vi "Day 7 - No Space Left On Device.vi"() -> ()   [LabVIEW 2020, in "AoC 2022.lvlib"]
uses:
  AoC 2022.lvlib
panel:
  in  "Directory Tree":string(tree)
  out "Puzzle Part-2 Answer":string
  out "Puzzle Answer":string
  in  "Puzzle Input":string="$ cd /\n$ ls\ndir a\n14848514 b.txt\n8504156 c.dat\ndir d\n$ cd a\n$ ls\ndir e\n29116 f\n2557 g\n62596 h.lst\n$ cd e\n$ ls\n584 i\n$ cd ..\n$ cd ..\n$ cd d\n$ ls\n4060174 j\n8033020 d.log\n5626152 d.ext\n7214296 k"
  # "Press Ctrl+M & Enter the Puzzle Input and run the VI"
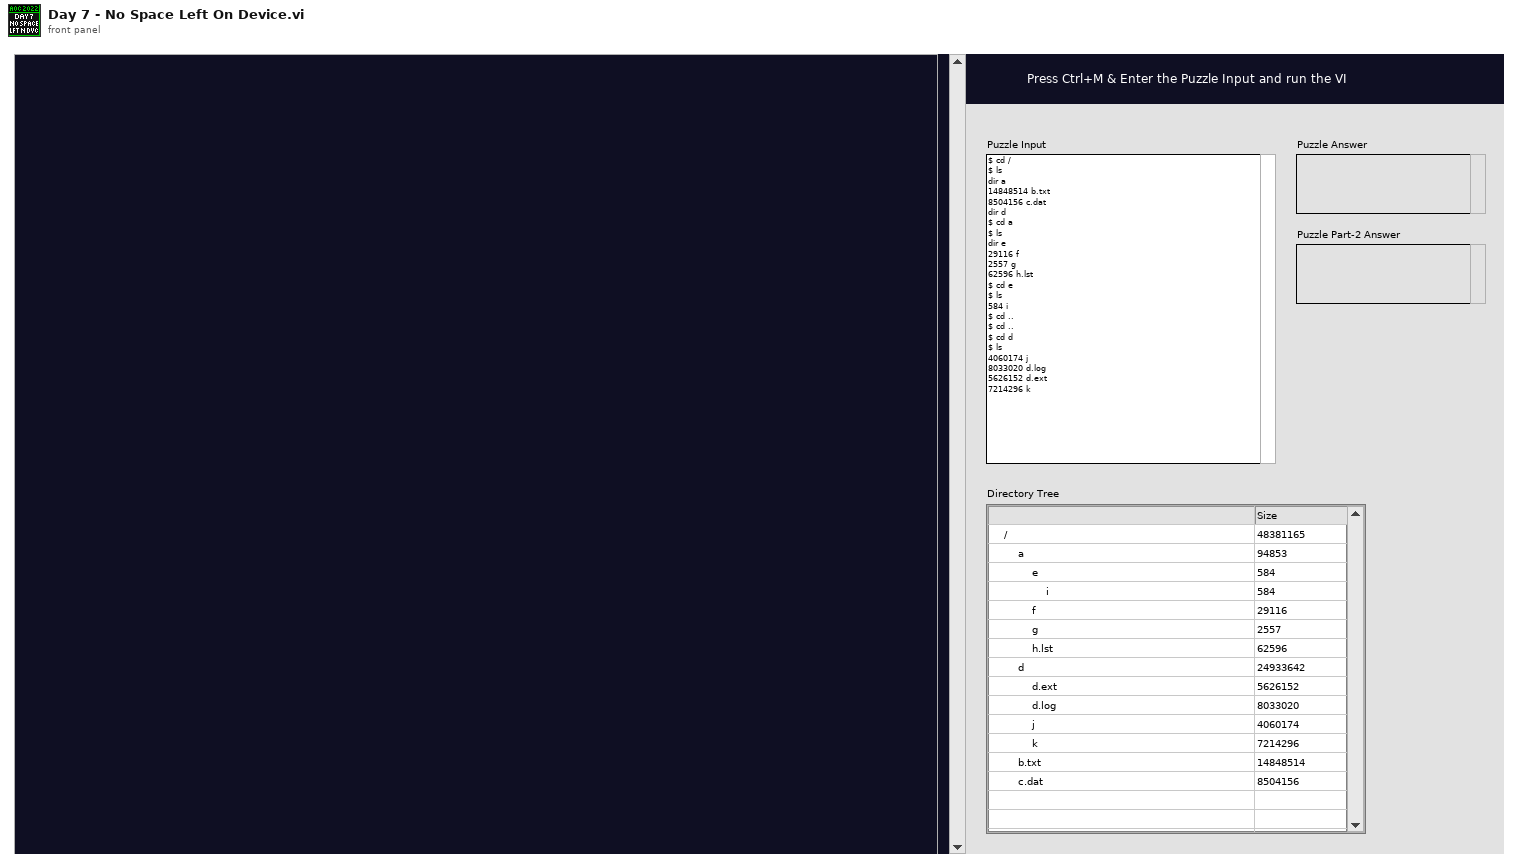
[diagram p1: front panel]
types:
  T1 = typedef "AoC 2022.lvlib/Directory Tree.ctl" = map{string, T2}
  T2 = typedef "AoC 2022.lvlib/Directory Content.ctl" = cluster{"Directories":set{string}, "Files":T3}
  T3 = typedef "AoC 2022.lvlib/File.ctl" = map{string, u64}
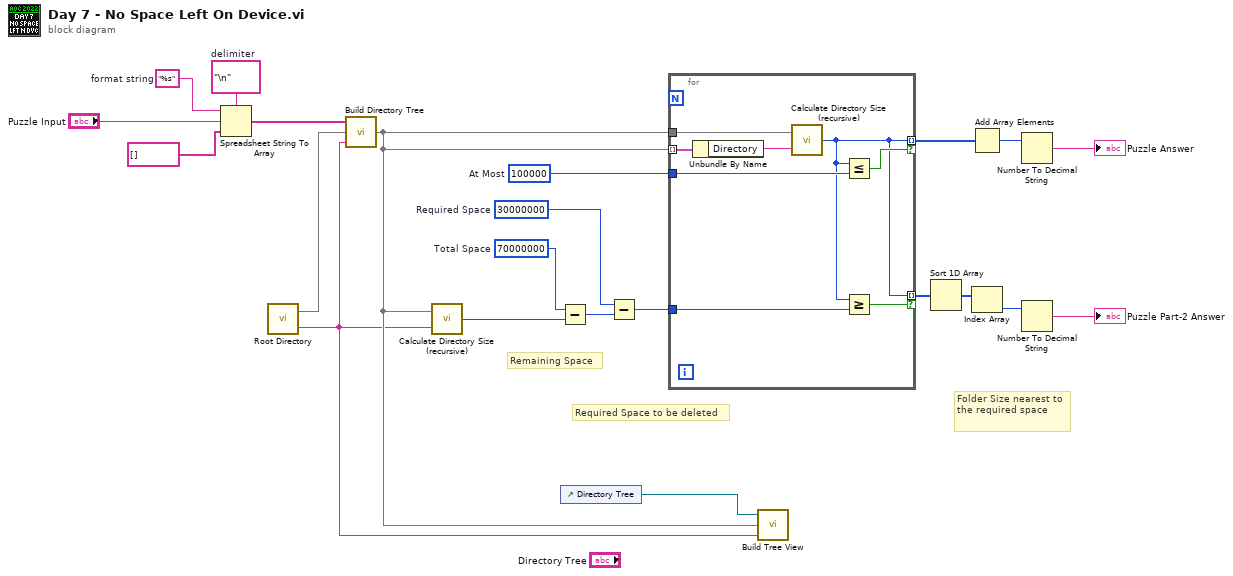
[diagram p0: block diagram]
diagram:
  w8 = u64 30000000  # Required Space
  w10 = u64 70000000  # Total Space
  w14 = u64 100000  # At Most
  w20 = "%s"  # format string
  w22 = "\n"  # delimiter
  # "Folder Size nearest to the required space"
  # "Required Space to be deleted"
  # "Remaining Space"
  n1 = Spreadsheet String To Array(delimiter (Tab)=w22, format string=w20, spreadsheet string="Puzzle Input", array type (2D Dbl)=string[] []) -> (array=w15:string[])
  n2 = call "Root Directory.vi"() -> ("Root Directory"=w1:string, "Directory Tree"=w16:T1)
  n3 = call "Build Directory Tree.vi"("Root Directory"=w1, "Directory Tree in"=w16, "Printed Data on Terminal"=w15) -> ("Directory Tree out"=w2:T1)  [unwired: 2 in]
  n4 = call "Calculate Directory Size (recursive).vi"("Directory"=w1, "Directory Tree"=w2) -> ("Directory Size"=w9:u64)
  n5 = Subtract(x=w10, y=w9) -> (x-y=w7:u64)
  n6 = control-ref of="Directory Tree"() -> (w3:refnum<vi>)
  n7 = Subtract(x=w8, y=w7) -> (x-y=w6:u64)
  n8 = for {
    tunnel: w2 -> [w30] mode=indexing
    tunnel: w2 -> [w28]
    tunnel: [w24] -> w11 mode=indexing if=w27
    tunnel: w14 -> [w26]
    tunnel: w6 -> [w25]
    tunnel: [w24] -> w5 mode=indexing if=w23
    n9 = Unbundle By Name(w30) -> ("Directory"=w29:string)
    n10 = call "Calculate Directory Size (recursive).vi"("Directory"=w29, "Directory Tree"=w28) -> ("Directory Size"=w24:u64)
    n11 = Less Or Equal?(x=w24, y=w26) -> (x <= y?=w27:bool)
    n12 = Greater Or Equal?(x=w24, y=w25) -> (x >= y?=w23:bool)
  }
  n13 = call "Build Tree View.vi"("Root Directory"=w1, "Directory Tree in"=w2, "TreeControl in"=w3) -> ()
  n14 = Sort 1D Array(array=w5) -> (sorted array=w4:u64[])
  n15 = Add Array Elements(numeric array=w11) -> (sum=w18:u64)
  n16 = Index Array(array=w4) -> (element=w13:u64)  [unwired: 1 in]
  n17 = Number To Decimal String(number=w18) -> (decimal integer string=→"Puzzle Answer":string)  [unwired: 1 in]
  n18 = Number To Decimal String(number=w13) -> (decimal integer string=→"Puzzle Part-2 Answer":string)  [unwired: 1 in]
